vi "Add Rows (String).vi"(7 "image path":path, 8 "error in (no error)":errorcluster, 9 "String Data":string[][](array[string]), 11 "DataTable in":refnum<class "DataTable.lvclass">) -> (0 "error out":errorcluster, 3 "DataTable out":refnum<class "DataTable.lvclass">)   [LabVIEW 2016, in "DataGrid.lvlib" / "DataTable.lvclass"]
doc: "This allows any number of rows to be added to the datatable. The data must match the columns defined for the grid."
uses:
  <userlib>/LabVIEWdotNetDataGrid/source/DataTable/DataTable.lvclass
  <userlib>/LabVIEWdotNetDataGrid/source/DataTable/DataTable.lvclass/DataTable.ctl
  System.Data
  <userlib>/LabVIEWdotNetDataGrid/source/GridColumn/GridColumn.lvclass/GridColumn.ctl
  <userlib>/LabVIEWdotNetDataGrid/source/GridColumn/Read datatype.vi
  <userlib>/LabVIEWdotNetDataGrid/source/GridColumn/GridColumn.lvclass
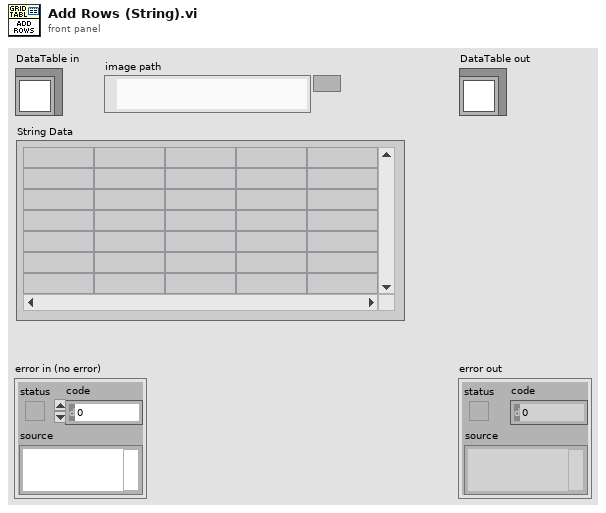
[diagram p1: front panel]
types:
  T1 = typedef "DataGrid.lvlib/GridColumn.lvclass/ColumnType.ctl" = enum16{"string", "image", "check", "numeric", "timestamp", "button", "combo", "link"}
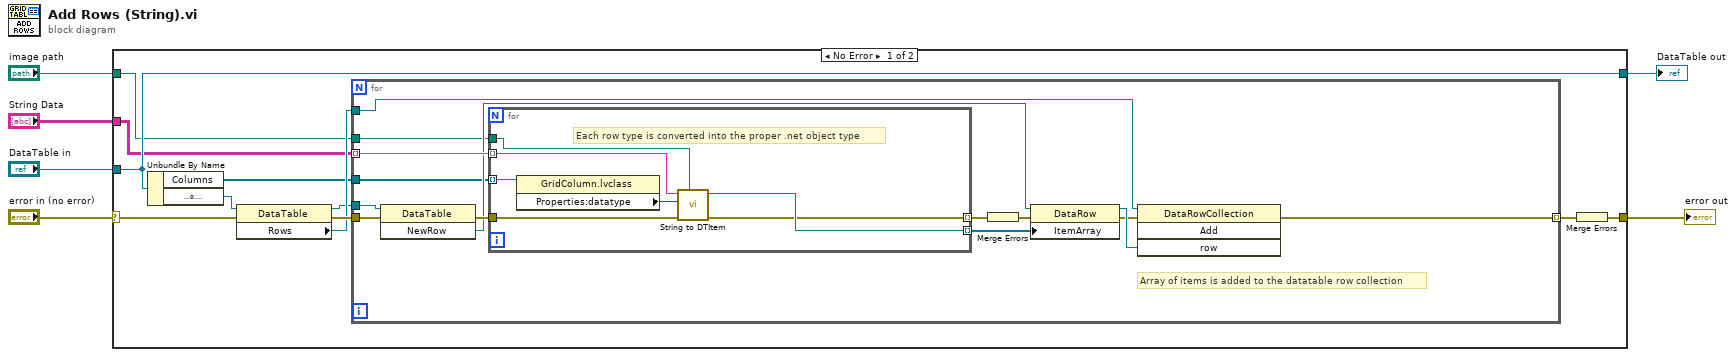
[diagram p0: block diagram]
diagram:
  n1 = case shown="No Error" "error in (no error)" {
    selector: "error in (no error)" -> [w13 w39]
    tunnel: [w14 w40] -> w4
    tunnel: "DataTable in" -> [w14 w40]
    tunnel: "String Data" -> [w12 _]
    tunnel: [w9 w39] -> w2
    tunnel: "image path" -> [w7 _]
    frame No Error {
      n2 = Unbundle By Name(w14) -> ("Columns"=w8:refnum<class "GridColumn.lvclass">[], "DataTable"=w11:refnum<k24>)
      n3 = property class="DataTable"(reference=w11, error in=w13) -> (reference out=w10:refnum<k24>, error out=w17:errorcluster, "Rows"=w16:refnum<k24>)
      n4 = for {
        tunnel: w16 -> [w30]
        tunnel: w10 -> [w31]
        tunnel: [w29] -> w15 mode=indexing
        tunnel: w12 -> [w28] mode=indexing
        tunnel: w17 -> [w20]
        tunnel: w8 -> [w19]
        tunnel: w7 -> [w18]
        # "Array of items is added to the datatable row collection"
        n5 = invoke class="DataTable" method="NewRow"(reference=w31, error in=w20) -> (error out=w27:errorcluster, "NewRow"=w26:refnum<k24>)  [unwired: 1 in, 1 out]
        n6 = for {
          tunnel: w28 -> [w33] mode=indexing
          tunnel: [w38] -> w24 mode=indexing
          tunnel: w27 -> [w37]
          tunnel: [w36] -> w23 mode=indexing
          tunnel: w19 -> [w35] mode=indexing
          tunnel: w18 -> [w34]
          # "Each row type is converted into the proper .net object type"
          n7 = property class="GridColumn.lvclass"(reference=w35) -> ("Properties:datatype"=w32:T1)  [unwired: 1 in, 2 out]
          n8 = call <userlib>:"String to DTItem.vi"("image path"=w34, "error in (no error)"=w37, "datatype"=w32, "element"=w33) -> ("error out"=w36:errorcluster, "DTItem .NET Refnum out"=w38:refnum<k24>)  [unwired: 6 in]
        }
        n9 = Merge Errors(w23) -> (w22:errorcluster)
        n10 = property class="DataRow"(reference=w26, error in=w22, "ItemArray"=w24) -> (reference out=w25:refnum<k24>, error out=w21:errorcluster)
        n11 = invoke class="DataRowCollection" method="Add"(reference=w30, error in=w21, "row"=w25) -> (error out=w29:errorcluster)  [unwired: 1 in, 3 out]
      }
      n12 = Merge Errors(w15) -> (w9:errorcluster)
    }
    frame Error {
    }
  }
  "error out" <- w2
  "DataTable out" <- w4
